vi "Sett_UP_Convert.vi"(8 "error in (no error)":errorcluster, 9 "Divider(1)":dbl=1.0, 11 "ISO 14443 A UP in":refnum<class "ISO 14443 A UP.lvclass">) -> (0 "error out":errorcluster, 2 "Waveform":waveform(dbl), 3 "ISO 14443 A UP out":refnum<class "ISO 14443 A UP.lvclass">)   [LabVIEW 2019, in "ISO 14443 A UP.lvclass"]
uses:
  ISO 14443 A UP.lvclass
  ISO 14443 A UP.lvclass/ISO 14443 A UP.ctl
  <vilib>/addons/Modulation/Analog/support/mod_Set Error Source.vi
  <vilib>/addons/Modulation/Digital/Support/Common/Validators/mod_Generate Filter Coefficients Validate.vi
  <vilib>/addons/Modulation/Digital/General/subVIs/mod_Generate Filter Coefficients.vi
  <vilib>/addons/Modulation/Digital/General/MT Generate ASK system parameters (M).vi
  <vilib>/addons/Modulation/niDMT.lvlib
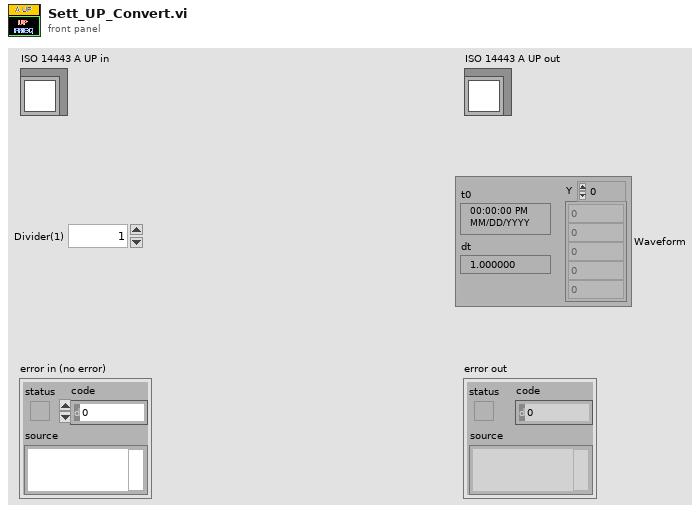
[diagram p1: front panel]
types:
  T1 = enum16{"none", "Raised Cosine", "Root Raised Cos", "Gaussian"}
  T2 = enum16{"FSK", "PSK", "QAM", "MSK", "PAM", "ASK", "CPM"}
  T3 = cluster{"samples per symbol (16)":i32, "symbol map":cdb[]}
  T4 = typedef "niAMT.lvlib/Complex Data Waveform.ctl" = cluster{"t0":dbl, "dt":dbl, "Y":cdb[]}
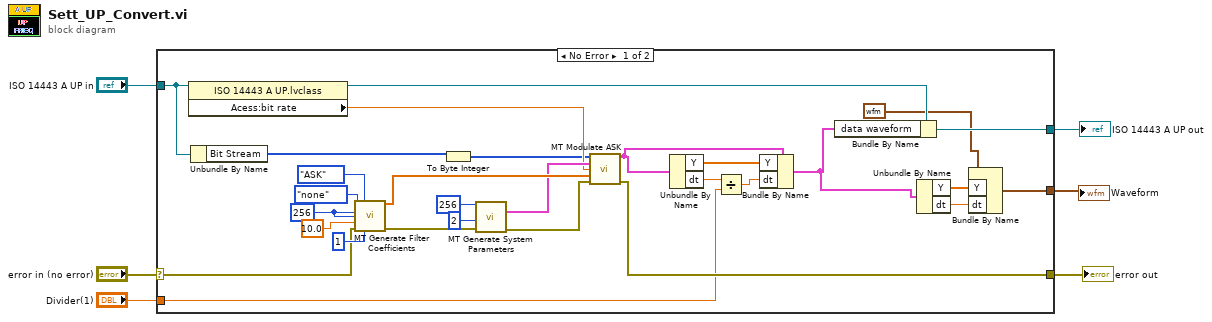
[diagram p0: block diagram]
diagram:
  n1 = case shown="No Error" "error in (no error)" {
    selector: "error in (no error)" -> [w22 w36]
    tunnel: [w20 w36] -> w5
    tunnel: "ISO 14443 A UP in" -> [w35 w37]
    tunnel: [w16 w37] -> w3
    tunnel: "Divider(1)" -> [w19 _]
    tunnel: [w8 _] -> w1
    frame No Error {
      w30 = 256 ("pulse shaping samples per symbol (16)")
      n2 = property class="ISO 14443 A UP.lvclass"(reference=w35) -> (reference out=w21:refnum<class "ISO 14443 A UP.lvclass">, "Acess:bit rate"=w23:dbl)  [unwired: 1 in, 1 out]
      n3 = Unbundle By Name(w35) -> ("Bit Stream"=w18:u8[])
      n4 = call <vilib>:"MT Generate Filter Coefficients.vi"("pulse shaping filter (none)"=T1."none", "modulation type"=T2."ASK", "pulse shaping samples per symbol (16)"=w30, "matched samples per symbol (16)"=w30, "filter parameter"=10.0, "error in (no error)"=w22, "filter length (symbols)"=1) -> ("pulse shaping filter coefficients"=w32:dbl[], "error out"=w27:errorcluster)  [unwired: 7 out]
      n5 = To Byte Integer(number=w18) -> (8bit integer=w17:i8[])
      n6 = call-poly <vilib>:"MT Generate System Parameters.vi"("samples per symbol (16)"=256, "M-ASK (2)"=2, "error in (no error)"=w27) -> ("ASK system parameters"=w24:T3, "error out"=w25:errorcluster)  [unwired: 11 out]
      n7 = call <vilib>:"MT Modulate ASK.vi"("input bit stream"=w17, "ASK system parameters"=w24, "symbol rate (Hz)"=w23, "pulse shaping filter coefficients"=w32, "error in (no error)"=w25) -> ("output complex waveform"=w12:T4, "error out"=w20:errorcluster)  [unwired: 8 in, 1 out]
      n8 = Unbundle By Name(w12) -> ("Y"=w13:cdb[], "dt"=w15:dbl)
      n9 = Divide(x=w15, y=w19) -> (x/y=w14:dbl)
      n10 = Bundle By Name(cluster=w12, "Y"=w13, "dt"=w14) -> (w9:T4)
      n11 = Bundle By Name(cluster=w21, "data waveform"=w9) -> (w16:refnum<class "ISO 14443 A UP.lvclass">)
      n12 = Unbundle By Name(w9) -> ("Y"=w11:cdb[], "dt"=w10:dbl)
      n13 = Bundle By Name(cluster=waveform(dbl) {"t0"=timestamp(0 s since 1904-01-01), "dt"=0.0, "Y"=array[8576 elements]} ("Waveform"), "Y"=w11, "dt"=w10) -> (w8:waveform(dbl))
    }
    frame Error {
    }
  }
  "error out" <- w5
  "ISO 14443 A UP out" <- w3
  "Waveform" <- w1
